vi "PlotBoat.vi"(6 "Heading":dbl, 7 "Trace Path":bool=TRUE, 8 "Bottum Right Pixel UTM":T1 {"North" format="%#_10f"; "East" format="%#_8f"}, 9 "Top Left Pixel UTM":T1 {"North" format="%#_10f"; "East" format="%#_8f"}, 10 "UTM Location":T1 {"North" format="%#_10f"; "East" format="%#_8f"}, 11 "Map in":T2) -> (2 "Boat Outside Img":bool, 3 "Map Out":T2)   [LabVIEW 2013]
uses:
  <vilib>/vision/Image Controls.llb/IMAQ Image.ctl
  trunk/Software/2-Think/2 Typedefs/UTM Location.ctl
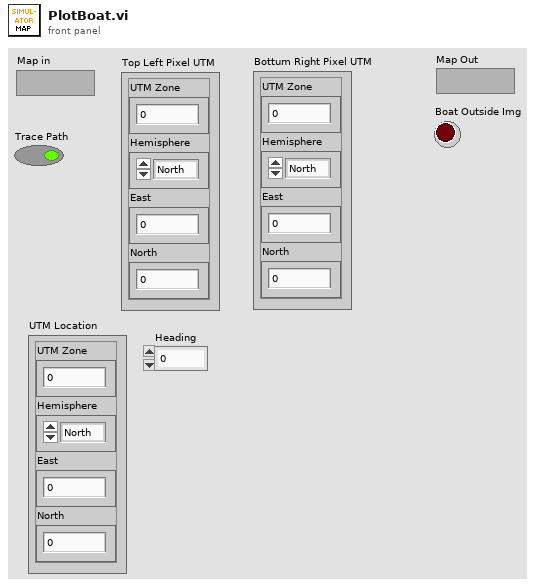
[diagram p1: front panel]
types:
  T1 = typedef "UTM Location.ctl" = cluster{"UTM Zone":dbl, "Hemisphere":enum16{"North", "South"}, "East":dbl, "North":dbl}
  T2 = typedef "IMAQ Image.ctl" = refnum<image>
  T3 = typedef "Overlay References.ctl" = cluster{"Boat Icon, Unroatated":T2, "Boat Icon, Rotated":T2, "Sail Icon, Unrotated":T2, "Sail Icon, Rotated":T2}
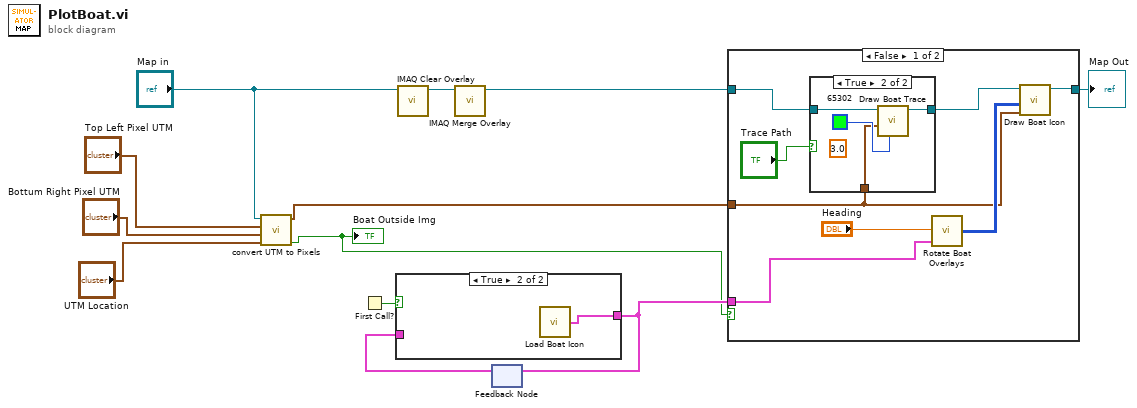
[diagram p0: block diagram]
diagram:
  n1 = call "convert UTM to Pixels.vi"("UTM position of Boat"="UTM Location", "Bottum Right Pixel UTM"="Bottum Right Pixel UTM", "Top Left Pixel UTM"="Top Left Pixel UTM", "Map in"="Map in") -> ("Boat Outside Img"=w2:bool, "Position"=w1:cluster{"X":i32, "Y":i32})  [unwired: 6 in]
  "Boat Outside Img" <- w2
  n2 = First Call?() -> (First Call?: T/F=w11:bool)
  n3 = call "IMAQ Clear Overlay"("Image"="Map in") -> ("Image Out"=w12:T2)  [unwired: 2 in, 8 out]
  n4 = call "IMAQ Merge Overlay"("Image Src"=w12) -> ("Image Dst Out"=w8:T2)  [unwired: 4 in, 6 out]
  n5 = feedback #1() -> (w9:T3)  [unwired: 1 in]
  n6 = case shown="True" w11 {
    tunnel: [w13 w14] -> w10
    tunnel: w9 -> [w13 _]
    frame False {
      # "image already\nloaded"
    }
    frame True {
      n7 = call "Load Boat Icon.vi"() -> ("Overlay References Out"=w14:T3)  [unwired: 1 in]
    }
  }
  n8 = feedback-in #1(w10) -> ()
  n9 = case shown="False" w2 {
    tunnel: [w20 w28] -> w7
    tunnel: w8 -> [w17 w28]
    tunnel: w10 -> [w21 _]
    tunnel: w1 -> [w16 _]
    frame False {
      n10 = case shown="True" "Trace Path" {
        tunnel: [w23 w26] -> w18
        tunnel: w17 -> [w23 w25]
        tunnel: w16 -> [_ w24]
        frame False {
        }
        frame True {
          (unwired) 3.0 ("Radius (px)")
          n11 = call "Draw Boat Trace.vi"("circle color"=u32 65302, "Position"=w24, "Image In"=w25) -> ("Image Out"=w26:T2)  [unwired: 8 in]
        }
      }
      n12 = call "Rotate Boat Overlays.vi"("Overlay References In"=w21, "Heading"="Heading") -> ("Rotated Boat Icon Bitmap Out"=w22:u32[][])  [unwired: 2 in, 1 out]
      n13 = call "Draw Boat Icon.vi"("Position"=w16, "Boat Bitmap"=w22, "Image In"=w18) -> ("Image Out"=w20:T2)  [unwired: 4 out]
    }
    frame True {
      # "don't draw\nif boat\noutside\nimage why not? lol jk"
    }
  }
  "Map Out" <- w7
